vi "Voltage to resistance.vi"(10 "data":dynamicdata(waveform), 11 "R2":dbl) -> (1 "Voltage 2":dbl, 2 "Numeric":dbl, 3 "Voltage 1":dbl)   [LabVIEW 2022 SP3]
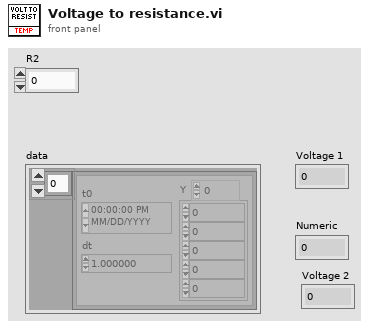
[diagram p1: front panel]
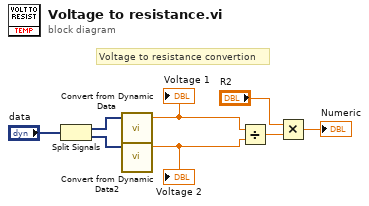
[diagram p0: block diagram]
diagram:
  # "Voltage to resistance convertion"
  n1 = Split Signals("data") -> (w2:dynamicdata, w3:dynamicdata)  [unwired: 2 in]
  n2 = call "Convert from Dynamic Data"("Dynamic Data Type"=w2) -> ("Scalar"=w4:dbl)  [unwired: 3 in]
  "Voltage 1" <- w4
  n3 = call "Convert from Dynamic Data2"("Dynamic Data Type"=w3) -> ("Scalar"=w5:dbl)  [unwired: 3 in]
  "Voltage 2" <- w5
  n4 = Divide(x=w4, y=w5) -> (x/y=w7:dbl)
  n5 = Multiply(x="R2", y=w7) -> (x*y=→"Numeric":dbl)
